vi "Write Waveforms to File (1D) with Advisory Dialog Control.vi"(6 "advisory dialog? (display:T)":bool, 8 "error in (no error)":errorcluster, 9 "append to file? (new file:F)":bool, 10 "waveform array":waveform(dbl)[](array[waveform]), 11 "file path (dialog if empty)":path) -> (0 "error out":errorcluster, 3 "new file path (Not A Path if cancelled)":path)   [LabVIEW 2010]
doc: "Creates a new file or appends to an existing file, writes the specified number of records to the file, then closes the file and checks for errors. Each record is an array of waveforms. Wire data to the <B>Waveform</B> input to determine the polymorphic instance to use or manually select the instance."
panel:
  # "CONTROL ABOVE ADDED"
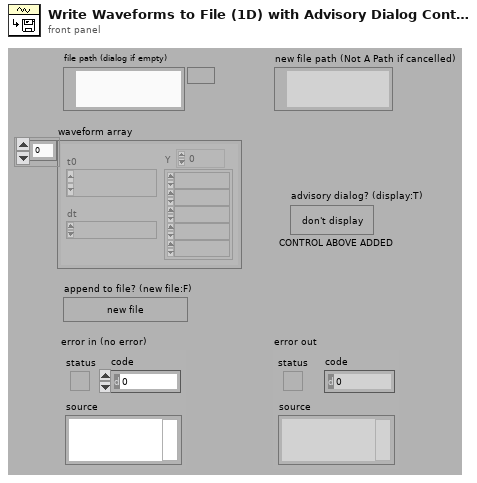
[diagram p1: front panel]
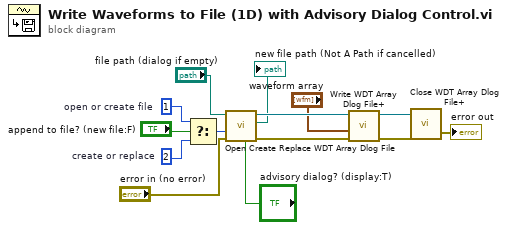
[diagram p0: block diagram]
diagram:
  w8 = i16 1  # open or create file
  w10 = i16 2  # create or replace
  n1 = Select(t=w8, s="append to file? (new file:F)", f=w10) -> (s? t:f=w7:i16)
  n2 = call <vilib>:"Open Create Replace WDT Array Dlog File.vi"("advisory dialog? (display:T)"="advisory dialog? (display:T)", "error in (not an error)"="error in (no error)", "function (open:0)"=w7, "file path"="file path (dialog if empty)") -> ("error out"=w14:errorcluster, "new file path"=→"new file path (Not A Path if cancelled)":path, "refnum"=w13:refnum<k1>)  [unwired: 4 in, 1 out]
  n3 = call <vilib>:"Write WDT Array Dlog File+.vi"("error in (no error)"=w14, "Array"="waveform array", "refnum"=w13) -> ("error out"=w11:errorcluster, "refnum"=w12:refnum<k1>)  [unwired: 6 in, 1 out]
  n4 = call <vilib>:"Close WDT Array Dlog File+.vi"("error in (no error)"=w11, "refnum"=w12) -> ("error out"=→"error out":errorcluster)  [unwired: 3 in, 2 out]
